vi "Lockin.DAQ.Create AO Tasks.vi"(8 "error in (no error)":errorcluster, 11 "Lockin.DAQ":refnum<class "Lockin.DAQ.lvclass">) -> (0 "error out":errorcluster, 3 "Lockin.DAQ":refnum<class "Lockin.DAQ.lvclass">)   [LabVIEW 2016, in "Lockin.DAQ.lvclass"]
uses:
  Lockin.DAQ.lvclass
  Lockin.DAQ.lvclass/Lockin.DAQ.ctl
  <vilib>/DAQmx/create/channels.llb/DAQmx Create Channel (AO-Voltage-Basic).vi
  <resource>/objmgr/daqmx.rc
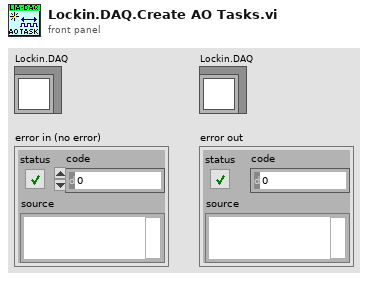
[diagram p1: front panel]
types:
  T1 = typedef "Lockin.DAQ.lvclass/AO.config-array.ctl" = T2[]
  T2 = typedef "Lockin.DAQ.lvclass/AO.config-cluster.ctl" = cluster{"AO.channels":tag, "AO.Range":T3, "output terminal configuration":i32, "DAQ Type":T4}
  T3 = typedef "Lockin.DAQ.lvclass/446xAO-enum.ctl" = enum16{"±0.1", "±1.0", "±10.0"}
  T4 = typedef "Lockin.DAQ.lvclass/DAQType-enum.ctl" = enum16{"None", "USB 4431", "PXI 446x"}
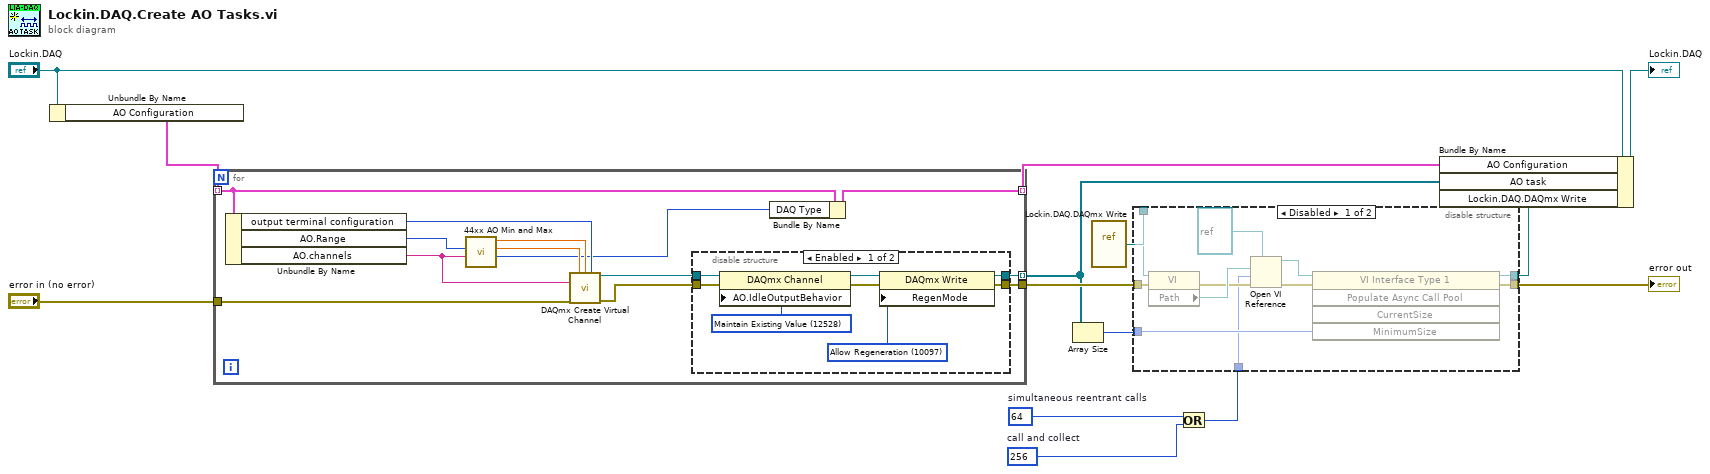
[diagram p0: block diagram]
diagram:
  w2 = 64  # simultaneous reentrant calls
  w3 = 256  # call and collect
  n1 = Unbundle By Name("Lockin.DAQ") -> ("AO Configuration"=w13:T1)
  n2 = for {
    tunnel: "error in (no error)" -> [w26]
    tunnel: [w16] -> w7
    tunnel: w13 -> [w15] mode=indexing
    tunnel: [w18] -> w11 mode=indexing
    tunnel: [w20] -> w5 mode=indexing
    n3 = Unbundle By Name(w15) -> ("output terminal configuration"=w22:i32, "AO.Range"=w21:T3, "AO.channels"=w23:tag)
    n4 = call "44xx AO Min and Max.vi"("AO.channels"=w23, "AO.Range"=w21) -> ("DAQ Type"=w19:T4, "AO.max"=w25:dbl, "AO.min"=w24:dbl)  [unwired: 7 in]
    n5 = call-poly <vilib>:"DAQmx Create Virtual Channel.vi"("maximum value"=w25, "minimum value"=w24, "output terminal configuration"=w22, "physical channels"=w23, "error in"=w26) -> ("task out"=w27:refnum<k21>, "error out"=w17:errorcluster)  [unwired: 9 in]
    n6 = disable-structure shown="Enabled" {
      disable-tunnel: w27 -> [w35 w37]
      disable-tunnel: [w32 w37] -> w20
      disable-tunnel: w17 -> [w31 w36]
      disable-tunnel: [w28 w36] -> w16
      frame Enabled {
        w29 = 10097 items=["Allow Regeneration"=10097, "Do Not Allow Regeneration"=10158] ("RegenMode")
        w30 = 12528 items=["Zero Volts"=12526, "High-Impedance"=12527, "Maintain Existing Value"=12528] ("AO.IdleOutputBehavior")
        n7 = property class="DAQmx Channel"(reference=w35, error in=w31, "AO.IdleOutputBehavior"=w30) -> (reference out=w34:refnum<k21>, error out=w33:errorcluster)
        n8 = property class="DAQmx Write"(reference=w34, error in=w33, "RegenMode"=w29) -> (reference out=w32:refnum<k21>, error out=w28:errorcluster)
      }
      frame Disabled {
      }
    }
    n9 = Bundle By Name(cluster=w15, "DAQ Type"=w19) -> (w18:T2)
  }
  n10 = Array Size(array=w5) -> (size(s)=w8:i32)
  n11 = vi-ref "Lockin.DAQ.DAQmx Write.vi"() -> (w9:refnum<vi>)
  n12 = Or(x=w2, y=w3) -> (x .or. y?=w1:i32)
  n13 = disable-structure shown="Disabled" {
    disable-tunnel: w9 -> [w48 _]
    disable-tunnel: w8 -> [w42 _]
    disable-tunnel: w7 -> [w41 w49]
    disable-tunnel: [w40 w49] -> w6
    disable-tunnel: [w39 _] -> w4
    disable-tunnel: w1 -> [w38 _]
    frame Disabled {
      n14 = property class="VI"(reference=w48, error in=w41) -> (error out=w46:errorcluster, "Path"=w47:path)  [unwired: 1 out]
      n15 = Open VI Reference(type specifier VI Refnum (for type only)=refnum<vi> refnum, vi path=w47, options=w38, error in (no error)=w46) -> (vi reference=w44:refnum<vi>, error out=w43:errorcluster)  [unwired: 2 in]
      n16 = invoke class="VI Interface Type 1" method="Populate Async Call Pool"(reference=w44, error in=w43, "MinimumSize"=w42) -> (reference out=w39:refnum<vi>, error out=w40:errorcluster)  [unwired: 2 in, 3 out]
    }
    frame Enabled {
    }
  }
  "error out" <- w6
  n17 = Bundle By Name(cluster="Lockin.DAQ", "AO Configuration"=w11, "AO task"=w5, "Lockin.DAQ.DAQmx Write"=w4) -> (→"Lockin.DAQ":refnum<class "Lockin.DAQ.lvclass">)
